vi "Write Invocation Request ID.vi"(8 "error in (no error)":errorcluster, 10 "Invocation Request ID":u64, 11 "Invocation Request in":refnum<class "Invocation Request ID.lvclass">) -> (0 "error out":errorcluster, 3 "Invocation Request out":refnum<class "Invocation Request ID.lvclass">)   [LabVIEW 2021, in "wamplv.lvlib" / "Invocation Request ID.lvclass"]
uses:
  Invocation Request ID.lvclass
  Invocation Request ID.lvclass/Invocation Request ID.ctl
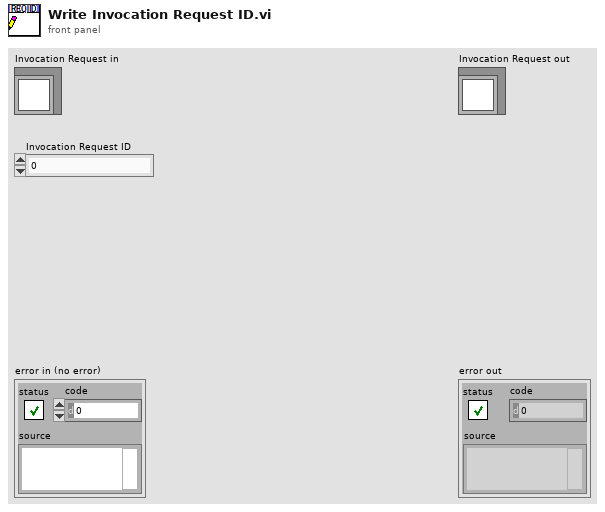
[diagram p1: front panel]
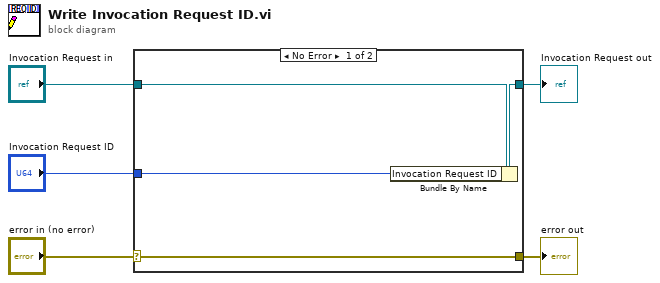
[diagram p0: block diagram]
diagram:
  n1 = case shown="No Error" "error in (no error)" {
    selector: "error in (no error)" -> [w9 w10]
    tunnel: [w9 w10] -> w4
    tunnel: [w7 w11] -> w2
    tunnel: "Invocation Request in" -> [w8 w11]
    tunnel: "Invocation Request ID" -> [w6 _]
    frame No Error {
      n2 = Bundle By Name(cluster=w8, "Invocation Request ID"=w6) -> (w7:refnum<class "Invocation Request ID.lvclass">)
    }
    frame Error {
    }
  }
  "error out" <- w4
  "Invocation Request out" <- w2
